vi "Insight_Send_Synch_Pulse_Power.vi"(6 "Atlas version major":i32, 8 "error in (no error)":errorcluster, 9 "Mode (Read / Write)":enum8{"Write", "Read"}(ring), 10 "Pwr Pulse Parameters":T1={"Amplitude"=1, "Delay (nsec)"=100.0, "Width (nsec)"=2.5, "Wavelength (nm)"=0.0}, 11 "telnet connection":T2) -> (0 "error out":errorcluster, 1 "response data":string, 2 "Pwr Pulse Parameters Out":T1, 3 "telnet  connection out":T2)   [LabVIEW 2011]
doc: "Insight Photonic Solutions\n\nThis VI generates a short optical power pulse from the laser, for use in synchronizing the laser sweep with a data acquisition system. This is a newer version of this synchronization pulse, which allows control over pulse amplitude, pulse delay and pulse width.\n\nInputs:\nRead/Write : query the pulse parameters or command the pulse to occur\nAmplitude : 1-10 (arbitrary units), controls the amplitude of the pulse.\nDelay (nsec) : 100 - 1000 nsec, default of 100 nsec.\nWidth (nsec) : 2.5 - 100 nsec, default 2.5 nsec.\n\nver 1.0 - original release\nver 3.3 - Parses response from Atlas version 3.2 and earlier, or Atlas version 3.3 and later"
uses:
  Telnet Session.ctl
  Pwr_pulse_parameters.ctl
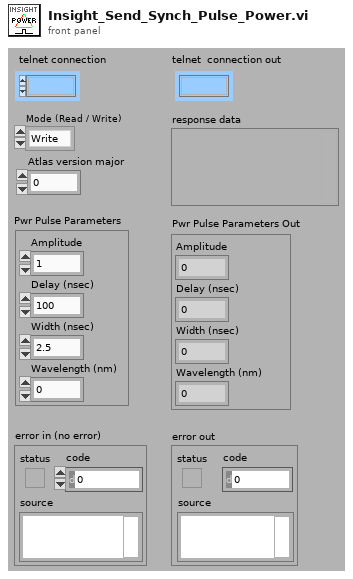
[diagram p1: front panel]
types:
  T1 = typedef "Pwr_pulse_parameters.ctl" = cluster{"Amplitude":i32, "Delay (nsec)":dbl, "Width (nsec)":dbl, "Wavelength (nm)":dbl}
  T2 = typedef "Telnet Session.ctl" = refnum<k1>
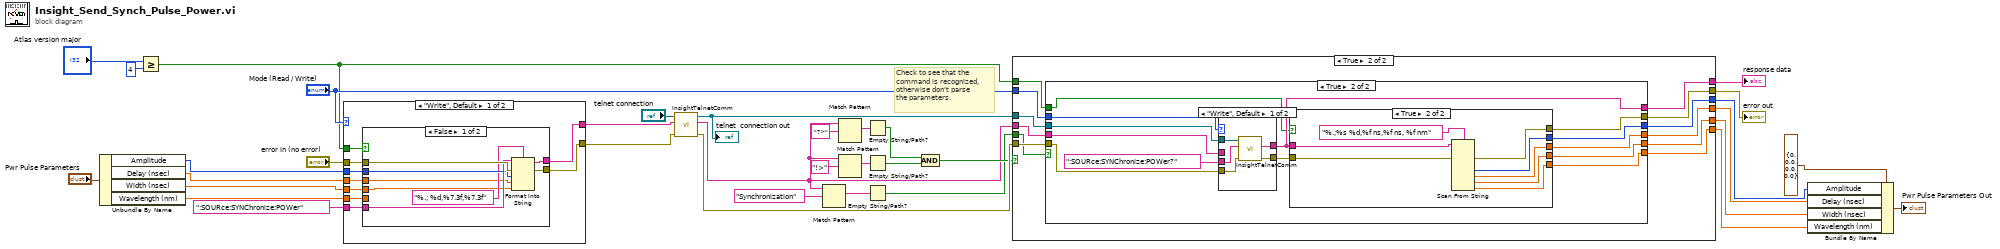
[diagram p0: block diagram]
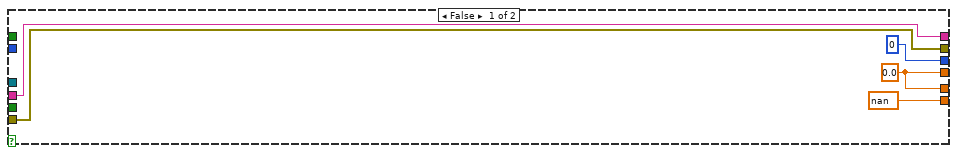
[diagram p2: hidden frame]
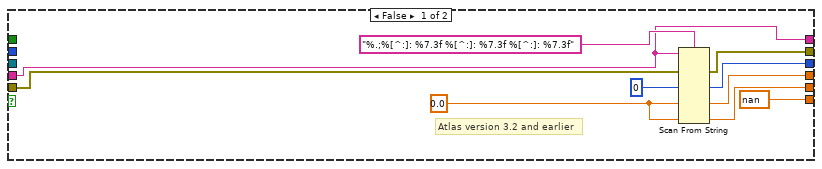
[diagram p3: hidden frame]
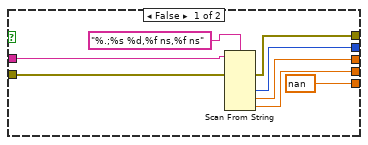
[diagram p4: hidden frame]
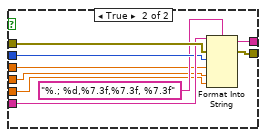
[diagram p6: hidden frame]
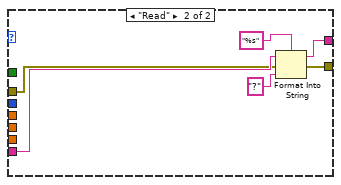
[diagram p7: hidden frame]
diagram:
  # "Check to see that the \ncommand is recognized,\notherwise don't parse \nthe parameters."
  n1 = Unbundle By Name("Pwr Pulse Parameters") -> ("Amplitude"=w24:i32, "Delay (nsec)"=w23:dbl, "Width (nsec)"=w22:dbl, "Wavelength (nm)"=w3:dbl)
  n2 = Greater Or Equal?(x="Atlas version major", y=4) -> (x >= y?=w1:bool)
  n3 = case shown="\"Write\", Default" "Mode (Read / Write)" {
    tunnel: [w44 w63] -> w32
    tunnel: "error in (no error)" -> [w43 w62]
    tunnel: ":SOURce:SYNChronize:POWer" ("String") -> [w42 w65]
    tunnel: w24 -> [w41 _]
    tunnel: [w40 w64] -> w34
    tunnel: w23 -> [w39 _]
    tunnel: w22 -> [w38 _]
    tunnel: w3 -> [w37 _]
    tunnel: w1 -> [w36 _]
    frame "Write", Default {
      n4 = case shown="False" w36 {
        tunnel: [w52 w61] -> w44
        tunnel: w43 -> [w51 w60]
        tunnel: w42 -> [w50 w59]
        tunnel: w41 -> [w49 w58]
        tunnel: [w47 w56] -> w40
        tunnel: w39 -> [w46 w55]
        tunnel: w38 -> [w45 w54]
        tunnel: w37 -> [_ w53]
        frame False {
          n5 = Format Into String(format string="%.; %d,%7.3f,%7.3f", initial string=w50, error in=w51, w49, w46, w45) -> (resulting string=w47:string, error out=w52:errorcluster)
        }
        frame True {
          n6 = Format Into String(format string="%.; %d,%7.3f,%7.3f, %7.3f", initial string=w59, error in=w60, w58, w55, w54, w53) -> (resulting string=w56:string, error out=w61:errorcluster)
        }
      }
    }
    frame "Read" {
      n7 = Format Into String(format string="%s", initial string=w65, error in=w62, "?" ("input 1")) -> (resulting string=w64:string, error out=w63:errorcluster)
    }
  }
  n8 = call "InsightTelnetComm.vi"("error in"=w32, "write buffer (\"\")"=w34, "telnet connection"="telnet connection") -> ("error out"=w30:errorcluster, "response data"=w11:string, "telnet  connection out"=w10:T2)  [unwired: 4 in]
  "telnet  connection out" <- w10
  n9 = Match Pattern(string=w11, regular expression="Synchronization") -> (match substring=w16:string)  [unwired: 1 in, 3 out]
  n10 = Match Pattern(string=w11, regular expression="!>") -> (match substring=w27:string)  [unwired: 1 in, 3 out]
  n11 = Match Pattern(string=w11, regular expression="?>") -> (match substring=w28:string)  [unwired: 1 in, 3 out]
  n12 = Empty String/Path?(string/path=w28) -> (empty?=w14:bool)
  n13 = Empty String/Path?(string/path=w27) -> (empty?=w15:bool)
  n14 = Empty String/Path?(string/path=w16) -> (empty?=w9:bool)
  n15 = Compound Arithmetic op=AND(w14, w15) -> (w13:bool)
  n16 = case shown="True" w13 {
    tunnel: [0 ("default value 1") w84] -> w19
    tunnel: [w71 w83] -> w18
    tunnel: [w71 w82] -> w17
    tunnel: [w72 w81] -> w31
    tunnel: w30 -> [w72 w80]
    tunnel: w11 -> [w69 w79]
    tunnel: w9 -> [_ w78]
    tunnel: "Mode (Read / Write)" -> [_ w77]
    tunnel: w10 -> [_ w76]
    tunnel: [w69 w75] -> w8
    tunnel: [nan w74] -> w2
    tunnel: w1 -> [_ w73]
    frame False {
      w71 = 0.0 ("default value 1")
    }
    frame True {
      n17 = case shown="True" w78 {
        tunnel: [w91 w107] -> w84
        tunnel: [w90 w105] -> w83
        tunnel: [w89 w104] -> w82
        tunnel: [w88 w106] -> w81
        tunnel: w80 -> [w87 w103]
        tunnel: w79 -> [w86 w98]
        tunnel: w77 -> [_ w99]
        tunnel: w76 -> [_ w101]
        tunnel: [w86 w97] -> w75
        tunnel: [nan w96] -> w74
        tunnel: w73 -> [_ w95]
        frame False {
          w92 = 0.0 ("default value 1")
          # "Atlas version 3.2 and earlier"
          n18 = Scan From String(format string="%.;%[^:]: %7.3f %[^:]: %7.3f %[^:]: %7.3f", input string=w86, error in=w87, default 2=0 ("default value 1"), default 4=w92, default 6=w92) -> (error out=w88:errorcluster, output 2=w91:i32, output 4=w90:dbl, output 6=w89:dbl)  [unwired: 7 in, 2 out]
        }
        frame True {
          n19 = case shown="\"Write\", Default" w99 {
            tunnel: w103 -> [w128 w129]
            tunnel: [w127 w129] -> w102
            tunnel: w101 -> [w126 _]
            tunnel: ":SOURce:SYNChronize:POWer?" ("String") -> [w125 _]
            tunnel: w98 -> [_ w130]
            tunnel: [w124 w130] -> w97
            frame "Write", Default {
              n20 = call "InsightTelnetComm.vi"("error in"=w128, "write buffer (\"\")"=w125, "telnet connection"=w126) -> ("error out"=w127:errorcluster, "response data"=w124:string)  [unwired: 4 in, 1 out]
            }
            frame "Read" {
            }
          }
          n21 = case shown="True" w95 {
            tunnel: [w114 w122] -> w107
            tunnel: [w113 w121] -> w106
            tunnel: [w112 w120] -> w105
            tunnel: [w111 w119] -> w104
            tunnel: w102 -> [w110 w118]
            tunnel: w97 -> [w109 w117]
            tunnel: [nan w116] -> w96
            frame False {
              n22 = Scan From String(format string="%.;%s %d,%f ns,%f ns", input string=w109, error in=w110) -> (error out=w113:errorcluster, output 2=w114:i32, output 3=w112:dbl, output 4=w111:dbl)  [unwired: 6 in, 2 out]
            }
            frame True {
              n23 = Scan From String(format string="%.;%s %d,%f ns,%f ns, %f nm", input string=w117, error in=w118) -> (error out=w121:errorcluster, output 2=w122:i32, output 3=w120:dbl, output 4=w119:dbl, output 5=w116:dbl)  [unwired: 7 in, 2 out]
            }
          }
        }
      }
    }
  }
  "error out" <- w31
  "response data" <- w8
  n24 = Bundle By Name(cluster=T1 {"Amplitude"=0, "Delay (nsec)"=0.0, "Width (nsec)"=0.0, "Wavelength (nm)"=0.0} ("Pulse Parameters Out"), "Amplitude"=w19, "Delay (nsec)"=w18, "Width (nsec)"=w17, "Wavelength (nm)"=w2) -> (→"Pwr Pulse Parameters Out":T1)
